vi "Generate Data.vi"   [LabVIEW 2015, in "Global Data.lvlib"]
uses:
  Global Data.lvlib
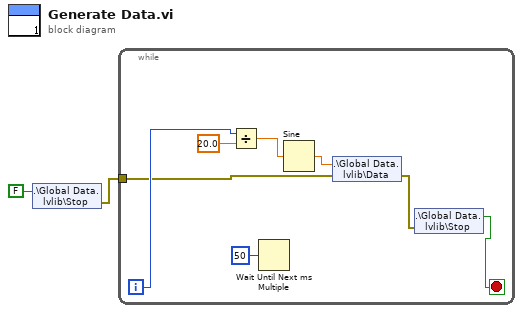
[diagram p0: block diagram]
diagram:
  n1 = shared-variable ".\\Global Data.lvlib\\Stop"(FALSE ("Stop")) -> (error out=w1:errorcluster)  [unwired: 1 in]
  n2 = while {
    tunnel: w1 -> [w5]
    i -> [w8]
    stop <- w3 stop-if-true
    n3 = Divide(x=w8, y=20.0) -> (x/y=w10:dbl)
    n4 = Wait Until Next ms Multiple(millisecond multiple=u32 50) -> ()  [unwired: 1 out]
    n5 = Sine(x=w10) -> (sin(x)=w6:dbl)
    n6 = shared-variable ".\\Global Data.lvlib\\Data"(w6, error in=w5) -> (error out=w4:errorcluster)
    n7 = shared-variable ".\\Global Data.lvlib\\Stop"(error in=w4) -> (w3:bool)  [unwired: 1 out]
  }
